vi "LED_Calc Resistance Values.vi"(0 "LED-Voltage Values":dbl[](array[numeric]), 1 "LED Output Voltage(Vo)":dbl format="%#_13g", 5 "LED Forward Resistance(Rd)":dbl format="%#_13g", 7 "LED Forward Voltage (Vf)":dbl format="%#_13g", 9 "LED Current (Io)":dbl format="%#_13g", 11 "error in":errorcluster, 12 "Max Resistance range":dbl format="%#_13g") -> (6 "Resistance Values":dbl[](array[numeric]), 10 "Set LED Current Limit?":bool, 15 "error out":errorcluster)   [LabVIEW 2021, in "start-up.lvlib"]
uses:
  start-up.lvlib
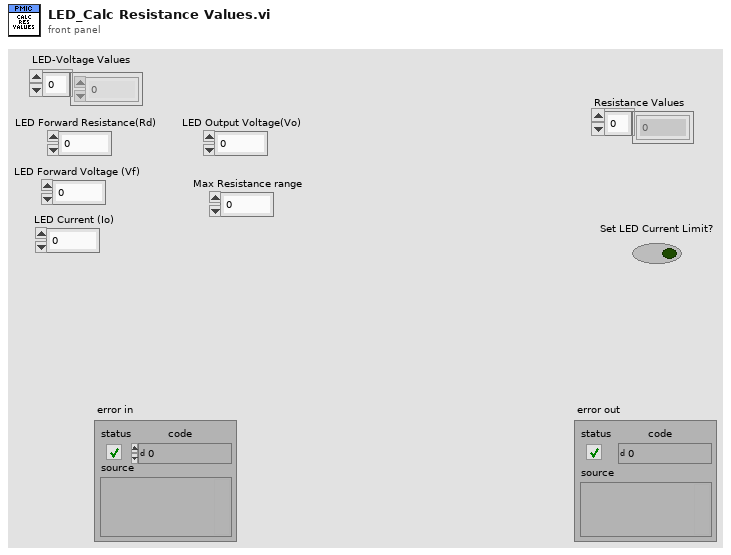
[diagram p1: front panel]
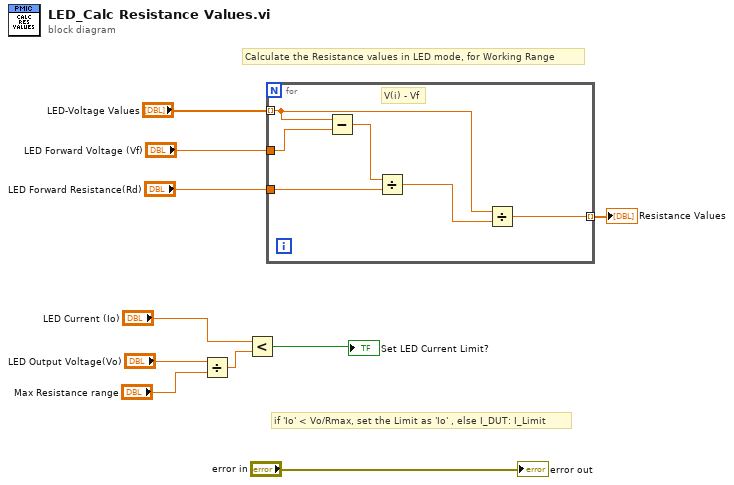
[diagram p0: block diagram]
diagram:
  # "if 'Io' < Vo/Rmax, set the Limit as 'Io' , else I_DUT: I_Limit"
  # "Calculate the Resistance values in LED mode, for Working Range"
  n1 = Divide(x="LED Output Voltage(Vo)", y="Max Resistance range") -> (x/y=w4:dbl)
  n2 = Less?(x="LED Current (Io)", y=w4) -> (x < y?=→"Set LED Current Limit?":bool)
  n3 = for {
    tunnel: "LED-Voltage Values" -> [w13] mode=indexing
    tunnel: "LED Forward Voltage (Vf)" -> [w16]
    tunnel: "LED Forward Resistance(Rd)" -> [w14]
    tunnel: [w12] -> w7 mode=indexing
    # "V(i) - Vf"
    n4 = Subtract(x=w13, y=w16) -> (x-y=w15:dbl)
    n5 = Divide(x=w15, y=w14) -> (x/y=w11:dbl)
    n6 = Divide(x=w13, y=w11) -> (x/y=w12:dbl)
  }
  "Resistance Values" <- w7
  "error out" <- "error in"
